vi "Move Files.vi"() -> ()   [LabVIEW 2011]
uses:
  OpenG.LIB/file/file.llb/Strip Path - Arrays__ogtk.vi
  OpenG.LIB/file/file.llb/Build Path - File Names Array__ogtk.vi
panel:
  in  "Start":bool
  out "Progress String":string
  out "Progress":dbl(slide) scale=0.0..1.0
  in  "Stop":bool
  out "Done":bool
  out "error out":errorcluster
  in  "Overwrite?":bool=TRUE
  in  "File Type Macro":string="*.tdms"
  in  "To Path":path
  in  "From Path":path
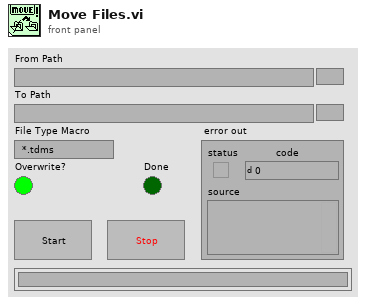
[diagram p1: front panel]
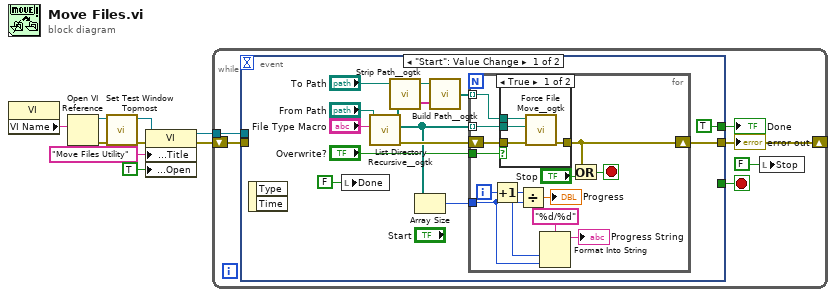
[diagram p0: block diagram]
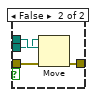
[diagram p2: hidden frame]
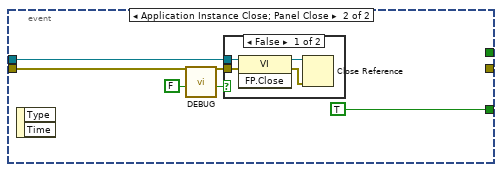
[diagram p3: hidden frame]
diagram:
  n1 = property class="VI"() -> ("VI Name"=w9:string)  [unwired: 2 in, 2 out]
  n2 = Open VI Reference(vi path=w9) -> (vi reference=w7:refnum<vi>, error out=w8:errorcluster)  [unwired: 1 in, 4 out]
  n3 = call "Set Test Window Topmost.vi"("error in (no error)"=w8, "VI Refnum"=w7) -> ("error out"=w5:errorcluster, "dup VI Refnum"=w6:refnum<vi>)  [unwired: 4 out]
  n4 = property class="VI"(reference=w6, error in=w5, "Front Panel Window:Title"="Move Files Utility", "Front Panel Window:Open"=TRUE) -> (reference out=w1:refnum<vi>, error out=w2:errorcluster)
  n5 = while {
    shift-right: [w12] -> _
    shift-left: w2 -> [w14]
    tunnel: w1 -> [w13]
    stop <- w15 stop-if-true
    n6 = event shown="[0] \"Start\": Value Change" {
      selector: _ -> [_ _]
      dyn-events: _ -> [_ _]
      timeout: _ -> [_ _]
      tunnel: [_ TRUE ("NewVal")] -> w15
      tunnel: [w18 _] -> w12
      tunnel: w14 -> [_ w51]
      tunnel: w13 -> [_ w50]
      tunnel: [TRUE ("Done") _] -> w11
      event "Start": Value Change {
        n7 = event-data() -> ()  [unwired: 1 in, 2 out]
        n8 = local write "Done"(FALSE ("Done")) -> ()
        n9 = call "List Directory Recursive__ogtk.vi"("pattern"="File Type Macro", "Path"="From Path") -> ("error out"=w27:errorcluster, "file paths"=w24:path[])  [unwired: 6 in, 2 out]
        n10 = call-poly "Strip Path__ogtk.vi"("path"=w24) -> ("name"=w26:string[])  [unwired: 1 out]
        n11 = Array Size(array=w24) -> (size(s)=w23:i32)
        n12 = call-poly "Build Path__ogtk.vi"("name or relative path"=w26, "base path"="To Path") -> ("appended path"=w25:path[])
        n13 = for {
          tunnel: w24 -> [w38] mode=indexing
          shift-right: [w34] -> w18
          shift-left: w27 -> [w40]
          tunnel: "Overwrite?" -> [w39]
          tunnel: w25 -> [w37] mode=indexing
          tunnel: w23 -> [w29]
          i -> [w33]
          stop <- w35 stop-if-true
          n14 = Increment(x=w33) -> (x+1=w30:i32)
          n15 = case shown="True" w39 {
            tunnel: w38 -> [w44 w45]
            tunnel: w40 -> [w43 w48]
            tunnel: [w42 w47] -> w34
            tunnel: w37 -> [w41 w46]
            frame True {
              n16 = call "Force File Move__ogtk.vi"("error in (no error)"=w43, "source"=w44, "target"=w41) -> ("error out"=w42:errorcluster)  [unwired: 3 in, 1 out]
            }
            frame False {
              n17 = Move(source path=w45, error in=w48, 10:w46) -> (error out=w47:errorcluster)  [unwired: 2 in, 2 out]
            }
          }
          n18 = Divide(x=w30, y=w29) -> (x/y=→"Progress":dbl)
          n19 = Format Into String(format string="%d/%d", w30, w29) -> (resulting string=→"Progress String":string)  [unwired: 2 in, 1 out]
          n20 = Or(x=w34, y="Stop") -> (x .or. y?=w35:bool)
        }
      }
      event Application Instance Close; Panel Close {
        n21 = event-data() -> ()  [unwired: 1 in, 2 out]
        n22 = call "DEBUG.vi"("Dev DEBUG? (f)"=FALSE) -> ("DEBUG?"=w53:bool)  [unwired: 1 in, 5 out]
        n23 = case shown="False" w53 {
          tunnel: w50 -> [w57 _]
          tunnel: w51 -> [w55 _]
          frame False {
            n24 = invoke class="VI" method="FP.Close"(reference=w57, error in=w55) -> (reference out=w56:refnum<vi>, error out=w54:errorcluster)  [unwired: 1 in, 1 out]
            n25 = Close Reference(reference=w56, error in (no error)=w54) -> ()  [unwired: 1 out]
          }
          frame True {
          }
        }
      }
    }
    "error out" <- w12
    "Done" <- w11
    n26 = local write "Stop"(FALSE ("Done")) -> ()
  }
